vi "Next VIP Version.vi"() -> (0 "error out":errorcluster, 3 "Next Version":string)   [LabVIEW 2020]
uses:
  <vilib>/xml/Load XML File.vi
  <vilib>/xml/Close Reference(Node).vi
  <vilib>/xml/NI_XML.lvlib
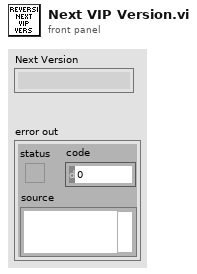
[diagram p1: front panel]
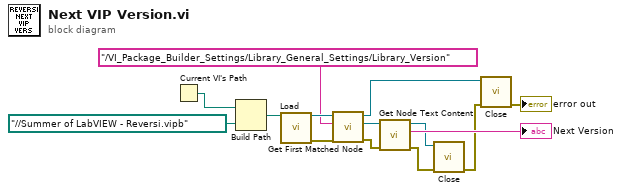
[diagram p0: block diagram]
diagram:
  n1 = Current VI's Path() -> (path=w1:path)
  n2 = Build Path(base path=w1, name or relative path=path "../../Summer of LabVIEW - Reversi.vipb") -> (appended path=w13:path)
  n3 = call-poly <vilib>:"Load.vi"("path to XML document"=w13) -> ("DOM document out"=w12:refnum<k20>, "error out"=w11:errorcluster)  [unwired: 12 in, 1 out]
  n4 = call <vilib>:"Get First Matched Node.vi"("error in (no error)"=w11, "XPath expression"="/VI_Package_Builder_Settings/Library_General_Settings/Library_Version", "node in"=w12) -> ("error out"=w8:errorcluster, "node result"=w9:refnum<k20>, "node out"=w4:refnum<k20>)  [unwired: 6 in]
  n5 = call <vilib>:"Get Node Text Content.vi"("error in (no error)"=w8, "node in"=w9) -> ("error out"=w5:errorcluster, "node text"=→"Next Version":string, "node out"=w6:refnum<k20>)  [unwired: 7 in]
  n6 = call-poly <vilib>:"Close.vi"("error in (no error)"=w5, "node"=w6) -> ("error out"=w3:errorcluster)  [unwired: 7 in]
  n7 = call-poly <vilib>:"Close.vi"("error in (no error)"=w3, "node"=w4) -> ("error out"=→"error out":errorcluster)  [unwired: 7 in]
